vi "SoftwarePWM.vi"() -> ()   [LabVIEW 2017]
panel:
  in  "Input":dbl
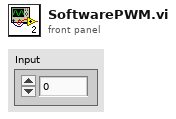
[diagram p1: front panel]
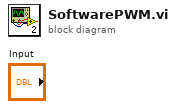
[diagram p0: block diagram]
diagram:
